vi "ToCommaSeparated.vi"(11 "Array":string[](array[string])) -> (3 "trimmed string":string)   [LabVIEW 2018, in "Matlab.lvclass"]
uses:
  Matlab.lvclass
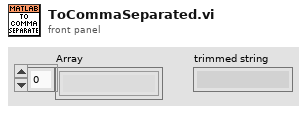
[diagram p1: front panel]
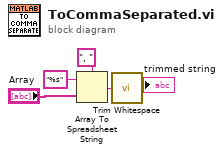
[diagram p0: block diagram]
diagram:
  n1 = Array To Spreadsheet String(delimiter (Tab)=", ", array="Array", 3:"%s" ("format string")) -> (spreadsheet string=w1:string)
  n2 = call <vilib>:"Trim Whitespace.vi"("string"=w1) -> ("trimmed string"=→"trimmed string":string)  [unwired: 1 in]
